vi "取任意长度数据.vi"() -> ()   [LabVIEW 2018]
panel:
  out "unsigned byte array[0]":u8
  out "元素":u16
  out "子数组":u16[](array[numeric])
  out "无符号字节数组":u8[](array[numeric])
  out "数组":u16[](array[numeric])
  out "size":i32
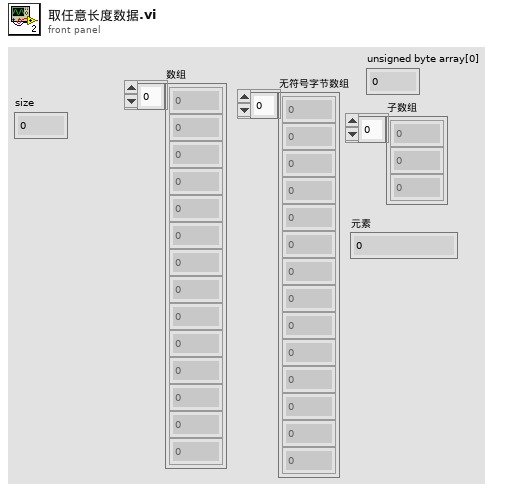
[diagram p1: front panel]
types:
  T1 = cluster{"unsigned byte array[0]":u8, "unsigned byte array[1]":u8, "unsigned byte array[2]":u8, "unsigned byte array[3]":u8, "unsigned byte array[4]":u8, "unsigned byte array[5]":u8, "unsigned byte array[6]":u8, "unsigned byte array[7]":u8, "unsigned byte array[8]":u8}
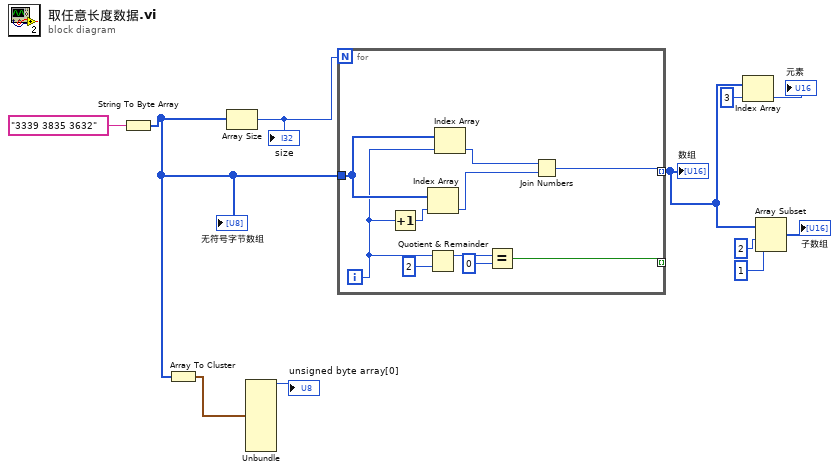
[diagram p0: block diagram]
diagram:
  n1 = String To Byte Array(string="3339 3835 3632" ("字符串")) -> (unsigned byte array=w3:u8[])
  "无符号字节数组" <- w3
  n2 = Array To Cluster(array=w3) -> (cluster=w2:T1)
  n3 = Array Size(array=w3) -> (size(s)=w10:i32)
  "size" <- w10
  n4 = Unbundle(w2) -> ("unsigned byte array[0]"=→"unsigned byte array[0]":u8)  [unwired: 8 out]
  n5 = for {
    N: w10 -> [_]
    tunnel: w3 -> [w21]
    tunnel: [w15] -> _ mode=indexing
    tunnel: [w12] -> w6 mode=indexing
    i -> [w19]
    n6 = Increment(x=w19) -> (x+1=w20:i32)
    n7 = Index Array(array=w21, index=w20) -> (element=w13:u8)
    n8 = Quotient & Remainder(x=w19, y=2) -> (x-y*floor(x/y)=w17:i32)  [unwired: 1 out]
    n9 = Index Array(array=w21, index=w19) -> (element=w14:u8)
    n10 = Equal?(x=w17, y=0) -> (x = y?=w15:bool)
    n11 = Join Numbers(hi=w14, lo=w13) -> ((hi.lo)=w12:u16)
  }
  "数组" <- w6
  n12 = Index Array(array=w6, index=3 ("索引")) -> (element=→"元素":u16)
  n13 = Array Subset(array=w6, index=2 ("索引"), length=1 ("长度")) -> (→"子数组":u16[])
